vi "Facade_Server.vi"(0 "Data In":T4, 2 "Display State In":T2, 3 "Container State":T3) -> (6 "Data Out":T4, 7 "Display State Out":T2, 8 "Action":T1)   [LabVIEW 2020, in "Server.xctl"]
uses:
  Server.xctl
  Data_Server.ctl
  <vilib>/_xctls/Container State.ctl
  State_Server.ctl
  <vilib>/_xctls/Action.ctl
  <vilib>/_xctls/XControlSupport.lvlib
panel:
  in  "Server":u16(ring)
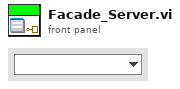
[diagram p1: front panel]
types:
  T1 = typedef "XControlSupport.lvlib/Action.ctl" = cluster{"Data Changed?":bool, "State Changed?":bool, "Action Name":string}
  T2 = typedef "Server.xctl/State_Server.ctl" = cluster{"Numeric":dbl}
  T3 = typedef "XControlSupport.lvlib/Container State.ctl" = cluster{"Indicator?":bool, "Run Mode?":bool, " Refnum":refnum<vi>}
  T4 = typedef "Server.xctl/Data_Server.ctl" = path
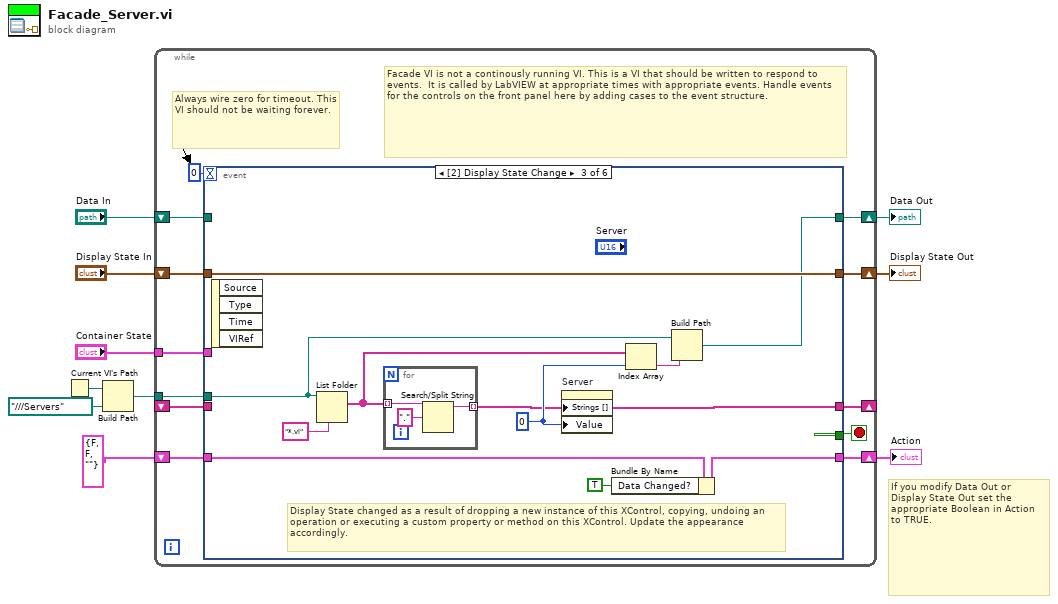
[diagram p0: block diagram]
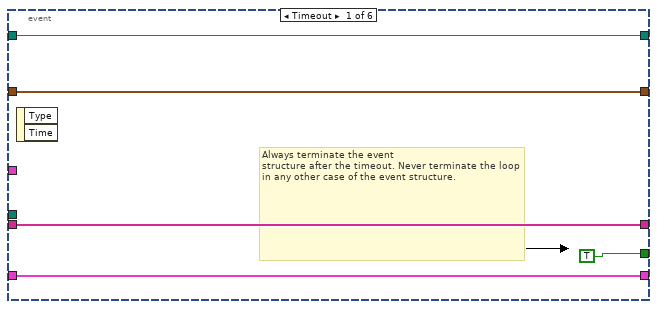
[diagram p2: hidden frame]
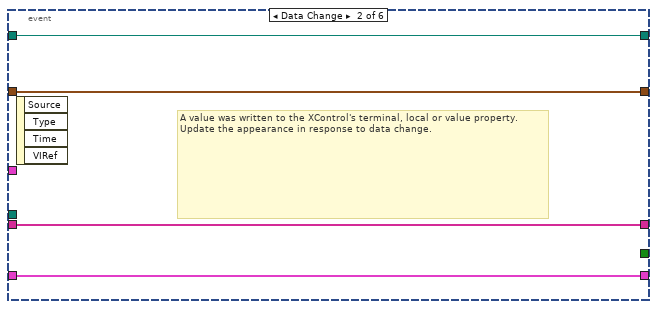
[diagram p3: hidden frame]
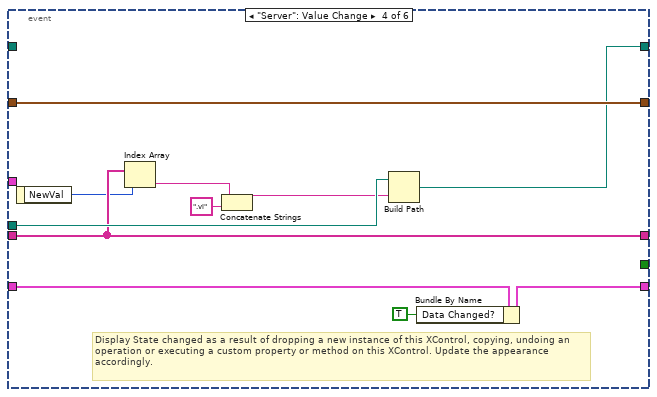
[diagram p4: hidden frame]
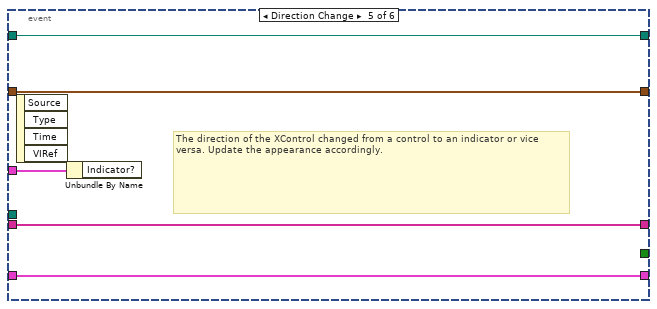
[diagram p5: hidden frame]
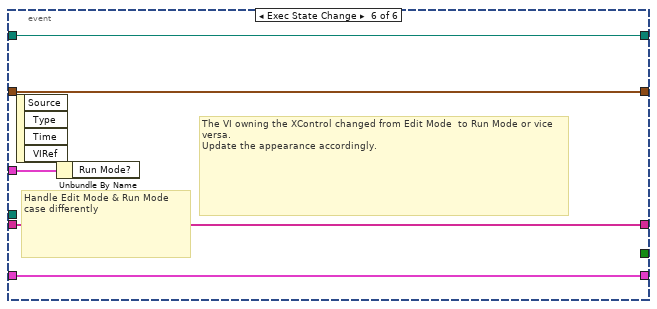
[diagram p6: hidden frame]
diagram:
  # "If you modify Data Out or\nDisplay State Out set the\nappropriate Boolean in Action\nto TRUE."
  n1 = Current VI's Path() -> (path=w3:path)
  n2 = Build Path(base path=w3, name or relative path=path "../../../Servers") -> (appended path=w1:path)
  n3 = while {
    shift-right: [w21] -> w7
    shift-left: "Display State In" -> [w22]
    tunnel: "Container State" -> [w18]
    shift-right: [w16] -> w10
    shift-left: "Data In" -> [w17]
    shift-right: [w14] -> w5
    shift-left: T1 {"Data Changed?"=FALSE, "State Changed?"=FALSE, "Action Name"=""} ("Action") -> [w15]
    tunnel: w1 -> [w13]
    shift-right: [w12] -> _
    shift-left: _ -> [w11]
    stop <- w20 stop-if-true
    # "Facade VI is not a continously running VI. This is a VI that should be written to respond to events.  It is called by LabVIEW at appropriate times with appropriate events. Handle events for the controls on the front panel here by adding cases to the event structure."
    # "Always wire zero for timeout. This\nVI should not be waiting forever."
    n4 = event shown="[2] Display State Change" {
      selector: _ -> [_ _ _ _ _ _]
      dyn-events: _ -> [_ _ _ _ _ _]
      timeout: 0 -> [_ _ _ _ _ _]
      tunnel: w22 -> [w25 w30 w42 w56 w60 w65]
      tunnel: [w25 w30 w42 w56 w60 w65] -> w21
      tunnel: [TRUE _ _ _ _ _] -> w20
      tunnel: w18 -> [_ _ _ _ w61 w66]
      tunnel: w17 -> [w24 w31 _ _ w59 w64]
      tunnel: [w24 w31 w38 w52 w59 w64] -> w16
      tunnel: [w26 w29 w39 w53 w58 w63] -> w14
      tunnel: w15 -> [w26 w29 w41 w55 w58 w63]
      tunnel: w13 -> [_ _ w37 w51 _ _]
      tunnel: [w23 w28 w33 w48 w57 w62] -> w12
      tunnel: w11 -> [w23 w28 _ w48 w57 w62]
      event Timeout {
        # "Always terminate the event\nstructure after the timeout. Never terminate the loop in any other case of the event structure."
        n5 = event-data() -> ()  [unwired: 1 in, 2 out]
      }
      event Data Change {
        # "A value was written to the XControl's terminal, local or value property.\nUpdate the appearance in response to data change."
        n6 = event-data() -> ()  [unwired: 1 in, 4 out]
      }
      event Display State Change {
        w34 = 0
        # "Display State changed as a result of dropping a new instance of this XControl, copying, undoing an operation or executing a custom property or method on this XControl. Update the appearance accordingly."
        n7 = event-data() -> ()  [unwired: 1 in, 4 out]
        n8 = List Folder(path=w37, pattern="*.vi") -> (filenames=w36:string[])  [unwired: 2 in, 3 out]
        n9 = for {
          tunnel: w36 -> [w45] mode=indexing
          tunnel: [w43] -> w33 mode=indexing
          n10 = Search/Split String(string=w45, search string/char (-)=".") -> (substring before match=w43:string)  [unwired: 1 in, 2 out]
        }
        n11 = property on="Server" class="Ring (strict)"("Strings []"=w33, "Value"=w34) -> ()  [unwired: 2 in, 2 out]
        n12 = Bundle By Name(cluster=w41, "Data Changed?"=TRUE) -> (w39:T1)
        n13 = Index Array(array=w36, index=w34) -> (element=w35:string)
        n14 = Build Path(base path=w37, name or relative path=w35) -> (appended path=w38:path)
      }
      event "Server": Value Change {
        # "Display State changed as a result of dropping a new instance of this XControl, copying, undoing an operation or executing a custom property or method on this XControl. Update the appearance accordingly."
        n15 = event-data() -> ("NewVal"=w47:u16)  [unwired: 1 in]
        n16 = Index Array(array=w48, index=w47) -> (element=w46:string)
        n17 = Concatenate Strings(w46, ".vi" ("string")) -> (w49:string)
        n18 = Build Path(base path=w51, name or relative path=w49) -> (appended path=w52:path)
        n19 = Bundle By Name(cluster=w55, "Data Changed?"=TRUE) -> (w53:T1)
      }
      event Direction Change {
        # "The direction of the XControl changed from a control to an indicator or vice versa. Update the appearance accordingly."
        n20 = event-data() -> ()  [unwired: 1 in, 4 out]
        n21 = Unbundle By Name(w61) -> ()  [unwired: 1 out]
      }
      event Exec State Change {
        # "The VI owning the XControl changed from Edit Mode  to Run Mode or vice versa.\nUpdate the appearance accordingly."
        # "Handle Edit Mode & Run Mode\ncase differently"
        n22 = event-data() -> ()  [unwired: 1 in, 4 out]
        n23 = Unbundle By Name(w66) -> ()  [unwired: 1 out]
      }
    }
  }
  "Display State Out" <- w7
  "Data Out" <- w10
  "Action" <- w5
